vi "DemoCDC.vi"() -> ()   [LabVIEW 2014]
uses:
  C:/Program Files (x86)/National Instruments/LabVIEW 2014/examples/Instrument IO/Serial/support/Serial - Settings.ctl
  <vilib>/Instr/_visa.llb/VISA Configure Serial Port (Instr).vi
panel:
  out "Distancia (cm)":i32(slide) scale=0.0..350.0
  in  "Grados":u64(knob)=30 max=180 step=5 scale=0.0..180.0
  in  "delay before read (ms)":u32=500
  in  "stop":bool
  in  "Serial Settings":T1={"baud rate"=9600, "data bits"=8, "parity"=enum."None", "stop bits"=10, "flow control"=0} {"flow control" items=["None"=0, "XON/XOFF"=1, "RTS/CTS"=2, "DTR/DSR"=4]; "stop bits" items=["1.0"=10, "1.5"=15, "2.0"=20]; "data bits" min=5 max=8 step=1; "baud rate" items=["75"=75, "110"=110, "134"=134, "150"=150, "300"=300, "600"=600, "1200"=1200, "1800"=1800, "2400"=2400, "4800"=4800, "7200"=7200, "9600"=9600, "14400"=14400, "19200"=19200, "28800"=28800, "38400"=38400, "56000"=56000, "57600"=57600, "115200"=115200, "128000"=128000, "230400"=230400]}
  in  "VISA resource name":refnum<visa-resource-name>="COM1"
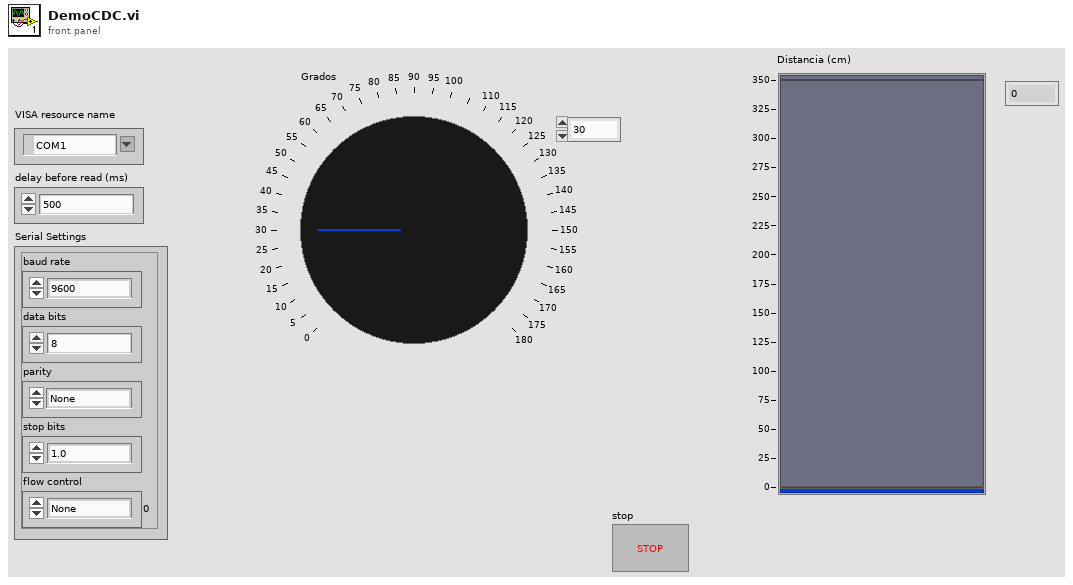
[diagram p1: front panel]
types:
  T1 = typedef "Serial - Settings.ctl" = cluster{"baud rate":u32, "data bits":u16, "parity":enum16{"None", "Odd", "Even", "Mark", "Space"}, "stop bits":u16, "flow control":u16}
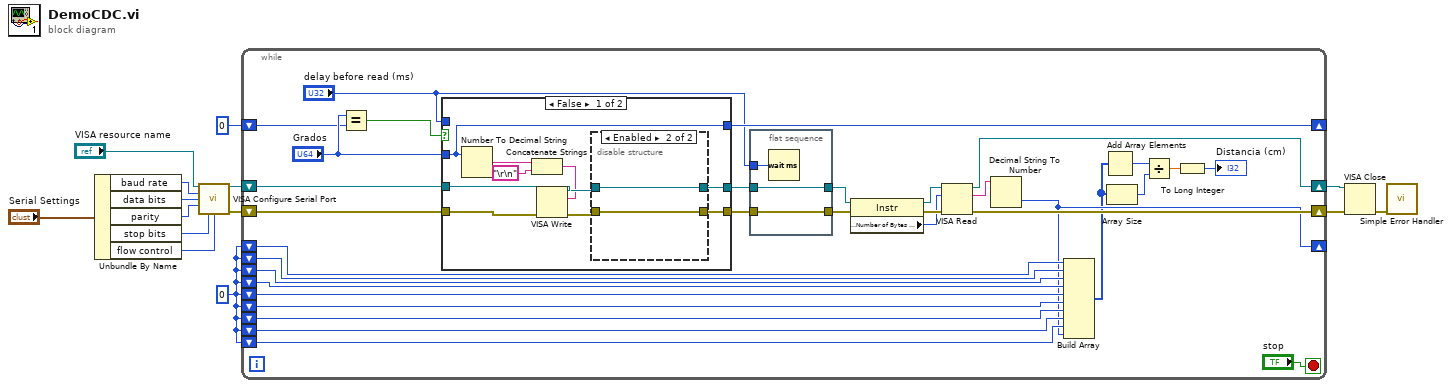
[diagram p0: block diagram]
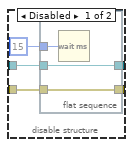
[diagram p2: hidden frame]
diagram:
  w1 = 0
  n1 = Unbundle By Name("Serial Settings") -> ("baud rate"=w7:u32, "data bits"=w6:u16, "parity"=w5:enum16{"None", "Odd", "Even", "Mark", "Space"}, "stop bits"=w4:u16, "flow control"=w3:u16)
  n2 = call-poly "VISA Configure Serial Port"("VISA resource name"="VISA resource name", "baud rate (9600)"=w7, "data bits (8)"=w6, "parity (0:none)"=w5, "stop bits (10: 1 bit)"=w4, "flow control (0:none)"=w3) -> ("VISA resource name out"=w12:refnum<visa-resource-name>, "error out"=w13:errorcluster)  [unwired: 3 in, 5 out]
  n3 = while {
    shift-right: [w47] -> w11
    shift-left: w13 -> [w37]
    shift-right: [w46] -> w10
    shift-left: w12 -> [w38]
    shift-right: [w36] -> _
    shift-left: u8 0 ("Dial") -> [w40]
    shift-right: [w20] -> _
    shift-left: w1 -> [w29]
    shift-left: w1 -> [w28]
    shift-left: w1 -> [w27]
    shift-left: w1 -> [w26]
    shift-left: w1 -> [w25]
    shift-left: w1 -> [w24]
    shift-left: w1 -> [w23]
    shift-left: w1 -> [w22]
    shift-left: w1 -> [w21]
    stop <- "stop" stop-if-true
    n4 = Equal?(x="Grados", y=w40) -> (x = y?=w39:bool)
    n5 = case shown="False" w39 {
      tunnel: "Grados" -> [w58 w71]
      tunnel: w38 -> [w60 w73]
      tunnel: w37 -> [w59 w72]
      tunnel: [w54 w72] -> w34
      tunnel: [w55 w73] -> w33
      tunnel: [w58 w71] -> w36
      tunnel: "delay before read (ms)" -> [_ _]
      frame False {
        n6 = Number To Decimal String(number=w58) -> (decimal integer string=w53:string)  [unwired: 1 in]
        n7 = Concatenate Strings(w53, "\r\n") -> (w52:string)
        n8 = VISA Write(VISA resource name=w60, write buffer=w52, error in (no error)=w59) -> (VISA resource name out=w56:refnum<visa-resource-name>, error out=w57:errorcluster)  [unwired: 1 out]
        n9 = disable-structure shown="Enabled" {
          disable-tunnel: w57 -> [w65 w69]
          disable-tunnel: w56 -> [w64 w70]
          disable-tunnel: [w63 w70] -> w55
          disable-tunnel: [w62 w69] -> w54
          frame Disabled {
            n10 = flat-sequence {
              tunnel: u32 15 ("delay before read (ms)") -> [w68]
              tunnel: w65 -> [w66]
              tunnel: w64 -> [w67]
              tunnel: [w67] -> w63
              tunnel: [w66] -> w62
              frame #0 {
                n11 = Wait (ms)(milliseconds to wait=w68) -> ()  [unwired: 1 out]
              }
            }
          }
          frame Enabled {
          }
        }
      }
      frame True {
      }
    }
    n12 = flat-sequence {
      tunnel: "delay before read (ms)" -> [w50]
      tunnel: w34 -> [w48]
      tunnel: w33 -> [w49]
      tunnel: [w49] -> w32
      tunnel: [w48] -> w31
      frame #0 {
        n13 = Wait (ms)(milliseconds to wait=w50) -> ()  [unwired: 1 out]
      }
    }
    n14 = property class="Instr"(reference=w32, error in=w31) -> (reference out=w45:refnum<visa-resource-name>, error out=w44:errorcluster, "Serial Settings:Number of Bytes at Serial Port"=w43:u32)
    n15 = VISA Read(VISA resource name=w45, byte count=w43, error in (no error)=w44) -> (VISA resource name out=w46:refnum<visa-resource-name>, read buffer=w35:string, error out=w47:errorcluster)  [unwired: 1 out]
    n16 = Decimal String To Number(string=w35) -> (number=w20:i32)  [unwired: 2 in, 1 out]
    n17 = Build Array(w29, w28, w27, w26, w25, w24, w23, w22, w21, w20) -> (w19:i32[])
    n18 = Add Array Elements(numeric array=w19) -> (sum=w18:i32)
    n19 = Array Size(array=w19) -> (size(s)=w17:i32)
    n20 = Divide(x=w18, y=w17) -> (x/y=w16:dbl)
    n21 = To Long Integer(number=w16) -> (32bit integer=→"Distancia (cm)":i32)
  }
  n22 = VISA Close(VISA resource name=w10, error in (no error)=w11) -> (error out=w9:errorcluster)
  n23 = call <vilib>:"Simple Error Handler.vi"("error in (no error)"=w9) -> ()  [unwired: 1 in, 8 out]
